vi "Go To Local.vi"(8 "error in (no error)":errorcluster, 11 "VISA resource name":refnum<visa-resource-name>) -> (0 "error out":errorcluster, 3 "VISA resource name out":refnum<visa-resource-name>)   [LabVIEW 2020, in "QuPMXdriver.lvlib"]
doc: "Set device to local mode. Enables the front panel push buttons if disabled."
uses:
  QuPMXdriver.lvlib
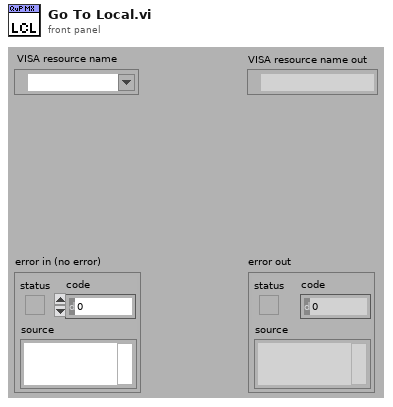
[diagram p1: front panel]
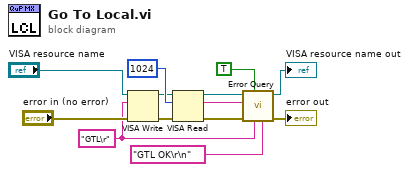
[diagram p0: block diagram]
diagram:
  w3 = "GTL\r"
  n1 = VISA Write(VISA resource name="VISA resource name", write buffer=w3, error in (no error)="error in (no error)") -> (VISA resource name out=w8:refnum<visa-resource-name>, error out=w1:errorcluster)  [unwired: 1 out]
  n2 = VISA Read(VISA resource name=w8, byte count=u32 1024, error in (no error)=w1) -> (VISA resource name out=w6:refnum<visa-resource-name>, read buffer=w2:string, error out=w5:errorcluster)  [unwired: 1 out]
  n3 = call "Error Query.vi"("Expected read buffer"="GTL OK\r\n" ("read buffer"), "Last command"=w3, "Ignore empty sequence? (T)"=TRUE, "error in (no error)"=w5, "Read buffer"=w2, "VISA resource name"=w6) -> ("error out"=→"error out":errorcluster, "VISA resource name out"=→"VISA resource name out":refnum<visa-resource-name>)  [unwired: 4 in]
